vi "Продбюсер-Консьюмер.vi"() -> ()   [LabVIEW 2021]
panel:
  in  "stop":bool
  in  "Хранилище":T1
  in  "Создать\n заказ":bool
  in  "Продьюсер":T2
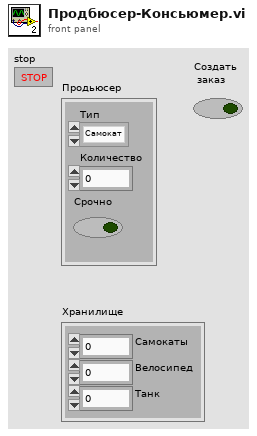
[diagram p1: front panel]
types:
  T1 = cluster{"Самокаты":dbl, "Велосипед":dbl, "Танк":dbl}
  T2 = typedef "Продьюсер.ctl" = cluster{"Срочно":bool, "Тип":enum16{"Самокат", "Велосипед", "Танк"}, "Количество":dbl}
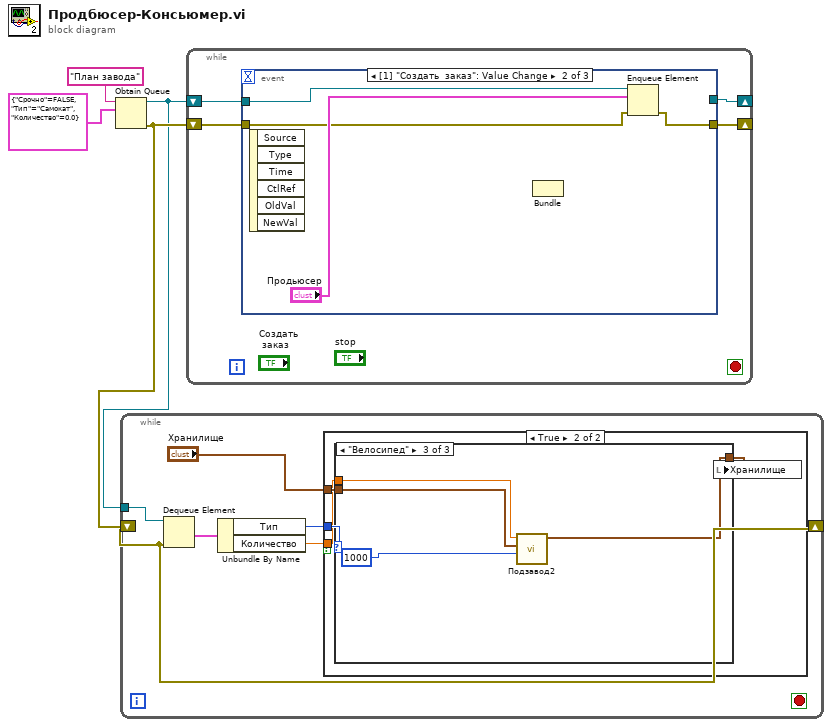
[diagram p0: block diagram]
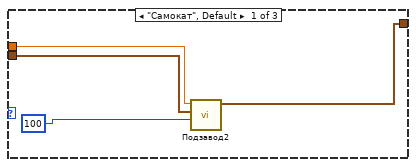
[diagram p3: hidden frame]
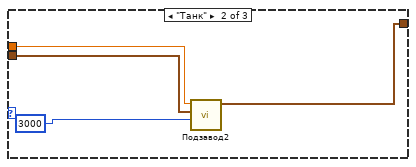
[diagram p4: hidden frame]
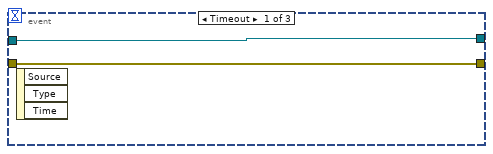
[diagram p5: hidden frame]
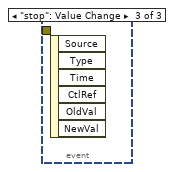
[diagram p6: hidden frame]
diagram:
  n1 = Obtain Queue(name (unnamed)="План завода", element data type=T2 {"Срочно"=FALSE, "Тип"=enum."Самокат", "Количество"=0.0} ("Продьюсер")) -> (queue out=w1:refnum<queue>, error out=w2:errorcluster)  [unwired: 3 in, 1 out]
  n2 = while {
    tunnel: w1 -> [w10]
    shift-right: [w5] -> _
    shift-left: w2 -> [w5]
    stop <- _ stop-if-true
    n3 = Dequeue Element(queue=w10, error in (no error)=w5) -> (element=w9:T2)  [unwired: 1 in, 3 out]
    n4 = Unbundle By Name(w9) -> ("Тип"=w8:enum16{"Самокат", "Велосипед", "Танк"}, "Количество"=w6:dbl)
    n5 = case shown="True" {
      selector: _ -> [_ _]
      tunnel: w8 -> [_ w14]
      tunnel: "Хранилище" -> [_ w13]
      tunnel: w6 -> [_ w12]
      frame False {
      }
      frame True {
        n6 = case shown="\"Велосипед\"" w14 {
          tunnel: w13 -> [w18 w22 w26]
          tunnel: w12 -> [w15 w19 w23]
          tunnel: [w17 w21 w25] -> w11
          frame "Самокат", Default {
            n7 = call "Подзавод2.vi"("milliseconds to wait"=u32 100, "Хранилище in"=w18, "Количество"=w15) -> ("Хранилище out"=w17:T1)  [unwired: 8 in]
          }
          frame "Танк" {
            n8 = call "Подзавод2.vi"("milliseconds to wait"=u32 3000, "Хранилище in"=w22, "Количество"=w19) -> ("Хранилище out"=w21:T1)  [unwired: 8 in]
          }
          frame "Велосипед" {
            n9 = call "Подзавод2.vi"("milliseconds to wait"=u32 1000, "Хранилище in"=w26, "Количество"=w23) -> ("Хранилище out"=w25:T1)  [unwired: 8 in]
          }
        }
        n10 = local write "Хранилище"(w11) -> ()
      }
    }
  }
  n11 = while {
    shift-right: [w28] -> _
    shift-left: w2 -> [w30]
    shift-right: [w27] -> _
    shift-left: w1 -> [w29]
    stop <- _ stop-if-true
    n12 = event shown="[1] \"Создать  заказ\": Value Change" {
      selector: _ -> [_ _ _]
      dyn-events: _ -> [_ _ _]
      timeout: _ -> [_ _ _]
      tunnel: w30 -> [w32 w33 _]
      tunnel: w29 -> [w31 w36 _]
      tunnel: [w32 w34 _] -> w28
      tunnel: [w31 _ _] -> w27
      event Timeout {
        n13 = event-data() -> ()  [unwired: 1 in, 3 out]
      }
      event "Создать\n заказ": Value Change {
        n14 = event-data() -> ()  [unwired: 1 in, 6 out]
        n15 = Bundle() -> ()  [unwired: 3 in, 1 out]
        n16 = Enqueue Element(queue=w36, element="Продьюсер", error in (no error)=w33) -> (error out=w34:errorcluster)  [unwired: 1 in, 2 out]
      }
      event "stop": Value Change {
        n17 = event-data() -> ()  [unwired: 1 in, 6 out]
      }
    }
  }
